vi "Update bitfile.vi"(8 "error in (no error)":errorcluster, 9 "FPGA addon name":string="FPGA Addon", 10 "bitfile name":string="TestBitfile2.lvbitx", 11 "sysdef path in":path) -> (0 "error out":errorcluster, 2 "FPGA addon refnum out":T1=18446744073709551615 format="%.0x", 3 "sysdef path out":path)   [LabVIEW 2021, in "Bitfile Reload System Tests.lvclass"]
uses:
  Bitfile Reload System Tests.lvclass
  <vilib>/NI VeriStand/Custom Device API/Custom Device Item Ref.ctl
  APIs/Scripting API/Scripting API.lvlib
  Addon/Addon System Explorer/FPGA Addon System Explorer.lvlib
  <vilib>/NI VeriStand/Custom Device API/Custom Device API.lvlib
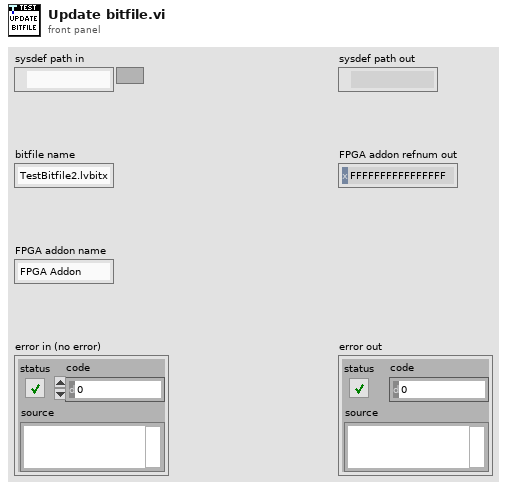
[diagram p1: front panel]
types:
  T1 = typedef "Custom Device API.lvlib/Custom Device Item Ref.ctl" = u64
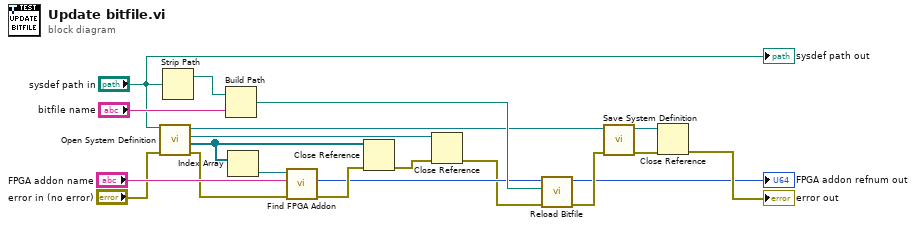
[diagram p0: block diagram]
diagram:
  n1 = call "Open System Definition.vi"("error in (no error)"="error in (no error)", "System Definition File"="sysdef path in") -> ("error out"=w6:errorcluster, "targets refnums"=w7:refnum<k24>[], "root refnum"=w8:refnum<k24>, "system definition refnum"=w2:refnum<k24>)  [unwired: 6 in]
  n2 = Strip Path(path="sysdef path in") -> (stripped path=w13:path)  [unwired: 1 out]
  n3 = Build Path(base path=w13, name or relative path="bitfile name") -> (appended path=w18:path)
  n4 = Index Array(array=w7) -> (element=w16:refnum<k24>)  [unwired: 1 in]
  n5 = call "Find FPGA Addon.vi"("error in"=w6, "FPGA addon name"="FPGA addon name", "target in"=w16) -> ("error out"=w19:errorcluster, "FPGA addon refnum out"=w14:T1)  [unwired: 5 in, 2 out]
  n6 = Close Reference(reference=w7, error in (no error)=w19) -> (error out=w12:errorcluster)
  n7 = Close Reference(reference=w8, error in (no error)=w12) -> (error out=w11:errorcluster)
  n8 = call "Reload Bitfile.vi"("error in (no error)"=w11, "NewVal"=w18, "Item Ref in"=w14) -> ("error out"=w5:errorcluster, "Section Ref out"=→"FPGA addon refnum out":T1)  [unwired: 7 in]
  n9 = call "Save System Definition.vi"("error in (no error)"=w5, ".NET Refnum in"=w2) -> ("error out"=w4:errorcluster, ".NET Refnum out"=w3:refnum<k24>)  [unwired: 8 in]
  n10 = Close Reference(reference=w3, error in (no error)=w4) -> (error out=→"error out":errorcluster)
  "sysdef path out" <- "sysdef path in"
